vi "Move Stage.vi"(8 "error in (no error)":errorcluster, 10 "Array":T1[](array[typedef]), 11 "MAS in":refnum<class "MAS.lvclass">) -> (0 "error out":errorcluster, 3 "MAS out":refnum<class "MAS.lvclass">)   [LabVIEW 2022 SP3, in "MAS.lvclass"]
uses:
  MAS.lvclass
  Axis New Value.ctl
  MAS.lvclass/MAS.ctl
  iMotion Controller/iMotion Controller.lvclass
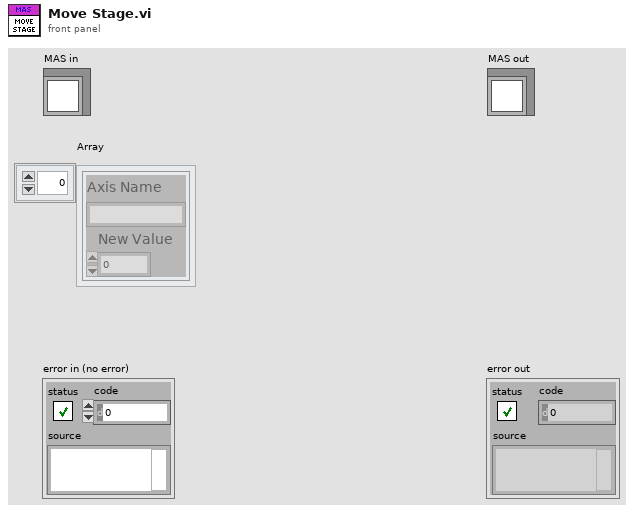
[diagram p1: front panel]
types:
  T1 = typedef "MAS.lvclass/Axis New Value.ctl" = cluster{"Axis Name":string, "New Value":dbl}
  T2 = map{string, refnum<class "iMotion Controller.lvclass">}
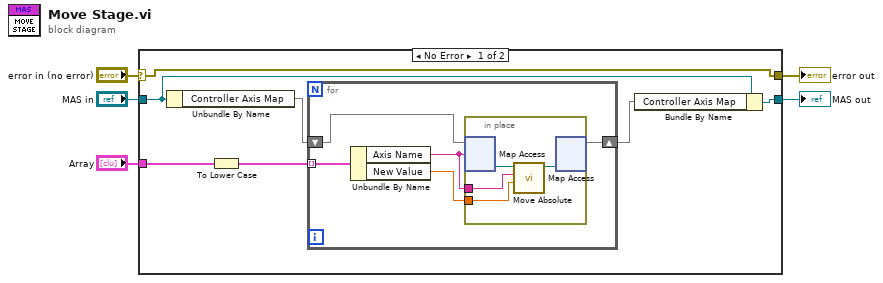
[diagram p0: block diagram]
diagram:
  n1 = case shown="No Error" "error in (no error)" {
    selector: "error in (no error)" -> [w12 w23]
    tunnel: [w12 w23] -> w4
    tunnel: [w8 w22] -> w2
    tunnel: "MAS in" -> [w10 w22]
    tunnel: "Array" -> [w11 _]
    frame No Error {
      n2 = Unbundle By Name(w10) -> ("Controller Axis Map"=w9:T2)
      n3 = To Lower Case(string=w11) -> (all lower case string=w6:T1[])
      n4 = for {
        tunnel: w6 -> [w17] mode=indexing
        shift-right: [w15] -> w7
        shift-left: w9 -> [w14]
        n5 = Unbundle By Name(w17) -> ("Axis Name"=w13:string, "New Value"=w16:dbl)
        n6 = in-place {
          in-place-border: w16 -> [w21]
          in-place-border: w13 -> [w20]
          n7 = in-place-map #1(w14, w13) -> (w19:refnum<class "iMotion Controller.lvclass">)  [unwired: 1 in, 1 out]
          n8 = call-dynamic "Move Absolute.vi"("Desired Position"=w21, "Axis Name"=w20, "iMotion Controller in"=w19) -> ("iMotion Controller out"=w18:refnum<class "iMotion Controller.lvclass">)  [unwired: 7 in, 1 out]
          n9 = in-place-map #1(w18) -> (w15:T2)  [unwired: 1 in, 2 out]
        }
      }
      n10 = Bundle By Name(cluster=w10, "Controller Axis Map"=w7) -> (w8:refnum<class "MAS.lvclass">)
    }
    frame Error {
    }
  }
  "error out" <- w4
  "MAS out" <- w2
